vi "LF Read File__ogtk.vi"   [LabVIEW 2017]
doc: "Reads data using a double precision number as offset to work for files larger than 2GB."
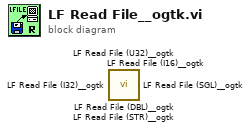
[diagram p0: block diagram]
diagram:
  n1 = call <userlib>:"LF Read File (DBL)__ogtk.vi"() -> ()  [unwired: 8 in, 4 out]
  n2 = call <userlib>:"LF Read File (I16)__ogtk.vi"() -> ()  [unwired: 8 in, 4 out]
  n3 = call <userlib>:"LF Read File (I32)__ogtk.vi"() -> ()  [unwired: 8 in, 4 out]
  n4 = call <userlib>:"LF Read File (SGL)__ogtk.vi"() -> ()  [unwired: 8 in, 4 out]
  n5 = call <userlib>:"LF Read File (STR)__ogtk.vi"() -> ()  [unwired: 8 in, 4 out]
  n6 = call <userlib>:"LF Read File (U32)__ogtk.vi"() -> ()  [unwired: 8 in, 4 out]
